vi "GA Open By IP.vi"(8 "error in (no error)":errorcluster caption="错误输入（无错误）", 10 "cCardIP":string, 11 "cPCIP":string) -> (0 "error out":errorcluster caption="错误输出", 1 "function return":i32, 2 "cCardIP out":string, 3 "cPCIP out":string)   [LabVIEW 2015, in "GAS.lvlib"]
doc: "extern \"C\" __declspec(dllimport) int GA_OpenByIP(char* cPCIP,char* cCardIP);"
uses:
  <userlib>/BP_GAS/GAS.lvlib
  <userlib>/BP_GAS/GAS.dll
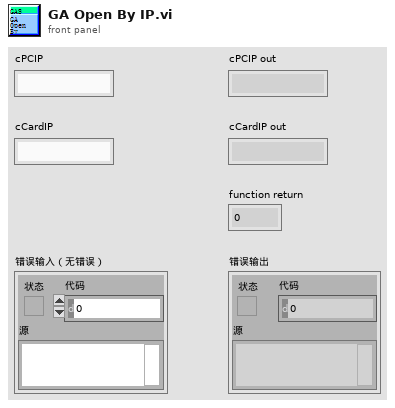
[diagram p1: front panel]
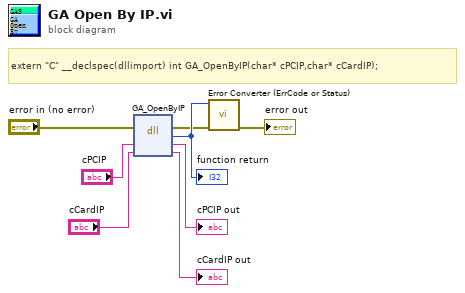
[diagram p0: block diagram]
diagram:
  # "extern \"C\" __declspec(dllimport) int GA_OpenByIP(char* cPCIP,char* cCardIP);"
  n1 = dll-call lib="E:/Program Files (x86)/National Instruments/LabVIEW 2015/user.lib/BP_GAS/GAS.*" fn="GA_OpenByIP"(error in="error in (no error)", "cPCIP"="cPCIP", "cCardIP"="cCardIP") -> (error out=w2:errorcluster, w8:i32, "cPCIP"=→"cPCIP out":string, "cCardIP"=→"cCardIP out":string)  [unwired: 2 in, 1 out]
  "function return" <- w8
  n2 = call "Error Converter (ErrCode or Status).vi"("error in (no error)"=w2, "error code"=w8) -> ("error out"=→"error out":errorcluster)  [unwired: 9 in]
